vi "GT_AlarmOn.vi"(2 "axis":i16, 3 "rtn_In":cluster{"rtn":i16, "Func":string}) -> (0 "axis out":i16, 1 "rtn_Out":cluster{"rtn":i16, "Func":string})   [LabVIEW 2014]
uses:
  VC6/gts.dll
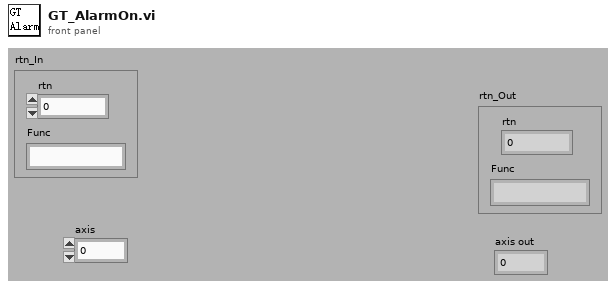
[diagram p1: front panel]
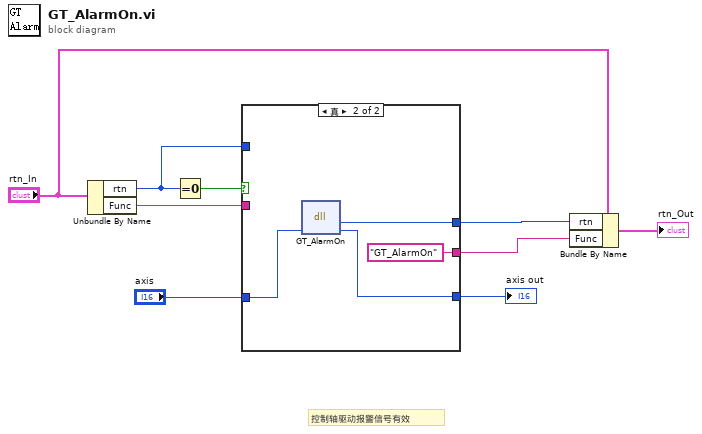
[diagram p0: block diagram]
diagram:
  # "控制轴驱动报警信号有效"
  n1 = Unbundle By Name("rtn_In") -> ("rtn"=w2:i16, "Func"=w8:string)
  n2 = Equal To 0?(x=w2) -> (x = 0?=w9:bool)
  n3 = case shown="真" w9 {
    tunnel: w8 -> [w11 _]
    tunnel: "axis" -> [w10 w16]
    tunnel: [w12 w15] -> w5
    tunnel: [w11 "GT_AlarmOn" ("Func")] -> w3
    tunnel: w2 -> [w12 _]
    tunnel: [w10 w13] -> w1
    frame False {
    }
    frame True {
      n4 = dll-call lib="PTH2Fabs DNewGTS AC-800LWin7版源程序-20170926gts85VC6gts.dll" fn="GT_AlarmOn"("axis"=w16) -> ("rtn"=w15:i16, "axis"=w13:i16)  [unwired: 3 in, 2 out]
    }
  }
  "axis out" <- w1
  n5 = Bundle By Name(cluster="rtn_In", "rtn"=w5, "Func"=w3) -> (→"rtn_Out":cluster{"rtn":i16, "Func":string})
